vi "MAIN_load_XY_positions.vi"(7 "XY positions":dbl[][](array[numeric]), 8 "error in":errorcluster, 9 "XY positions":refnum<vi>, 10 "ROI manager":i32(listbox), 11 "ROI manager":refnum<vi>) -> (0 "error out":errorcluster, 3 "Next task":T1, 4 "XY graph":cluster{dbl[], dbl[]}[](array[cluster]), 5 "XY positions OUT":dbl[][](array[numeric]))   [LabVIEW 2015]
uses:
  CONTROLS/Q_main_element.ctl
panel:
  in  "Start acquisition":bool
  out "XY positions":cluster{dbl[], dbl[]}[](graph)
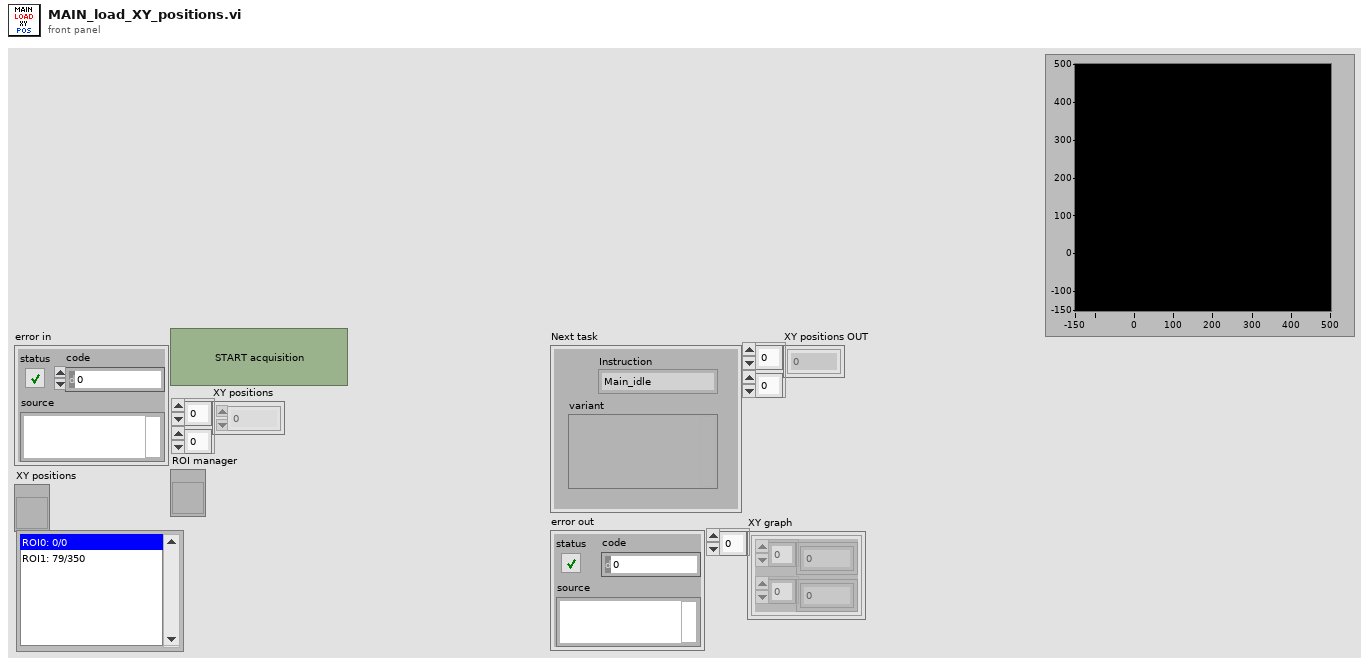
[diagram p1: front panel]
types:
  T1 = typedef "Q_main_element.ctl" = cluster{"variant":variant, "Instruction":enum16{"Main_idle", "Main_initialize", "Main_initialize_TDMS", "Main_initialize_Queue", "Main_error", "Main_DAQ_initialization_results", "Main_ASI_initialization_results", "Main_Piezo_initialization_results", "Main_Valve_initialization_results", "Main_Pump_initialization_results", "Main_CAMERA_initialization_results", "Main_FPGA_initialization_results", "Main_DAQ_error", "Main_ASI_error", "Main_Piezo_error", "Main_CAMERA_error", "Main_Valve_error", "Main_Pump_error", "Main_FPGA_error", "Main_start_acquiring", "Main_not_acquiring", "Main_acquiring", "Main_stop_acquiring", "Main_change_exposure", "Main_change_z_scan_parameters", "Main_define_ROI", "Main_define_mosaic", "Main_read_kinetic_time", "Main_cooler", "Main_read_temperature", "Main_save_XY", "Main_load_XY", "Main_discard_XY", "Main_move_to_XY", "Main_measure_QPD", "Main_autofocus_calibration", "Main_autofocus_initialization", "Main_autofocus_stop", "Main_save_PID", "Main_change_H_valve_position", "Main_two_way_valve", "Main_save_movie", "Main_init_single_scan", "Main_single_scan", "Main_stop_single_scan", "Main_merFISH_illumination_parameters", "Main_merFISH_buffer_probe_list", "Main_merFISH_injections_procedure", "Main_merFISH_save_setpoint", "Main_merFISH_DAPI_parameters", "Main_merFISH_Brightfield_parameters", "Main_merFISH_save_embryo_ROI", "Main_merFISH_init", "Main_merFISH_resume", "Main_merFISH_start_autofocus", "Main_merFISH_open_close_valve_merFISH", "Main_merFISH_open_close_valve_photobleaching", "Main_merFISH_hybridization", "Main_merFISH_move_to_ROI", "Main_merFISH_wait_stabilization", "Main_merFISH_move_to_REF", "Main_merFISH_scan", "Main_merFISH_photobleaching_injection", "Main_merFISH_photobleaching", "Main_merFISH_send_email", "Main_merFISH_close", "Main_STOP"}}
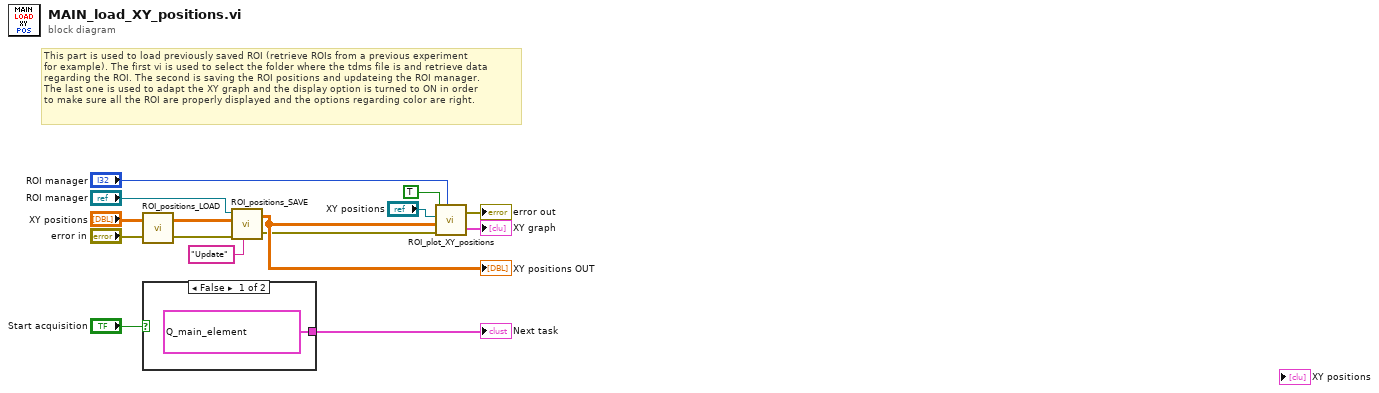
[diagram p0: block diagram]
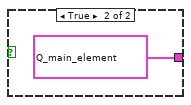
[diagram p2: hidden frame]
diagram:
  # "This part is used to load previously saved ROI (retrieve ROIs from a previous experiment\nfor example). The first vi is used to select the folder where the tdms file is and retrieve data\nregarding the ROI. The second is saving the ROI positions and updateing the ROI manager.\nThe last one is used to adapt the XY graph and the display option is turned to ON in order\nto make sure all the ROI are properly displayed and the options regarding color are right."
  n1 = call "ROI_positions_LOAD.vi"("error in"="error in", "XY positions"="XY positions") -> ("error out"=w11:errorcluster, "XY positions OUT"=w12:dbl[][])
  n2 = case shown="False" "Start acquisition" {
    tunnel: [T1 {"variant"=variant, "Instruction"=enum."Main_not_acquiring"} ("Q_main_element") T1 {"variant"=variant, "Instruction"=enum."Main_acquiring"} ("Q_main_element")] -> w7
    frame False {
    }
    frame True {
    }
  }
  "Next task" <- w7
  n3 = call "ROI_positions_SAVE.vi"("Choice"="Update", "XY positions"=w12, "error in"=w11, "ROI LstBox Refnum"="ROI manager") -> ("error out"=w13:errorcluster, "XY positions OUT"=w14:dbl[][])  [unwired: 2 in]
  "XY positions OUT" <- w14
  n4 = call "ROI_plot_XY_positions.vi"("Display?"=TRUE, "XYGraph Refnum"="XY positions", "XY positions"=w14, "error in"=w13, "ROI manager"="ROI manager") -> ("error out"=→"error out":errorcluster, "XY graph"=→"XY graph":cluster{dbl[], dbl[]}[])
